vi "From 1D String Tree Data.vi"(11 "Tree Data":refnum<class "Tree Data.lvclass">) -> (2 "1D String":string[](array[string]))   [LabVIEW 2017, in "Tree API.lvlib" / "1D String.lvclass"]
doc: "Extract a 1D String value from Tree Data type."
uses:
  1D String.lvclass
  Tree Data/Tree Data.lvclass
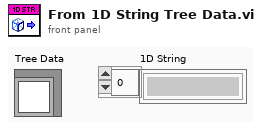
[diagram p1: front panel]
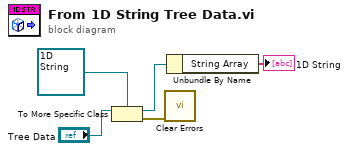
[diagram p0: block diagram]
diagram:
  n1 = To More Specific Class(target class=refnum<class "1D String.lvclass"> refnum ("StringArray.lvclass"), reference="Tree Data") -> (specific class reference=w3:refnum<class "1D String.lvclass">, error out=w4:errorcluster)  [unwired: 1 in]
  n2 = call <vilib>:"Clear Errors.vi"("error in (no error)"=w4) -> ()  [unwired: 5 in, 2 out]
  n3 = Unbundle By Name(w3) -> ("String Array"=→"1D String":string[])
